vi "SerialMgr.vi"(0 "VISA Resource Name":refnum<visa-resource-name>="COM1", 1 "baud rate (921600)":u32=921600, 2 "data bits (8)":u16=8 min=5 max=8 step=1, 3 "parity (0:none)":enum16{"None", "Odd", "Even", "Mark", "Space"}(ring), 4 "stop bits (10: 1 bit)":u16(ring)=10 items=["1.0"=10, "1.5"=15, "2.0"=20], 5 "flow control (0:None)":enum16{"None", "XON/XOFF", "RTS/CTS"}(ring)) -> ()   [LabVIEW 2016]
doc: "This VI is the solution to Exercise 9-5 of the LabVIEW Basics I Course.\n\nThis VI communicates through the serial port to the NI Instrument Simulator using the VISA functions."
uses:
  SndMsgType.ctl
  <vilib>/Instr/_visa.llb/VISA Configure Serial Port (Instr).vi
  GlobalVars.vi
panel:
  # "* VISA resource name control *"
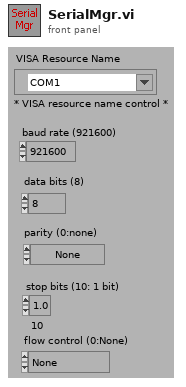
[diagram p1: front panel]
types:
  T1 = typedef "SndMsgType.ctl" = cluster{"Length":u16, "Formatted Msg":u8[]}
  T2 = typedef "Queue RefNum" = refnum<k1>
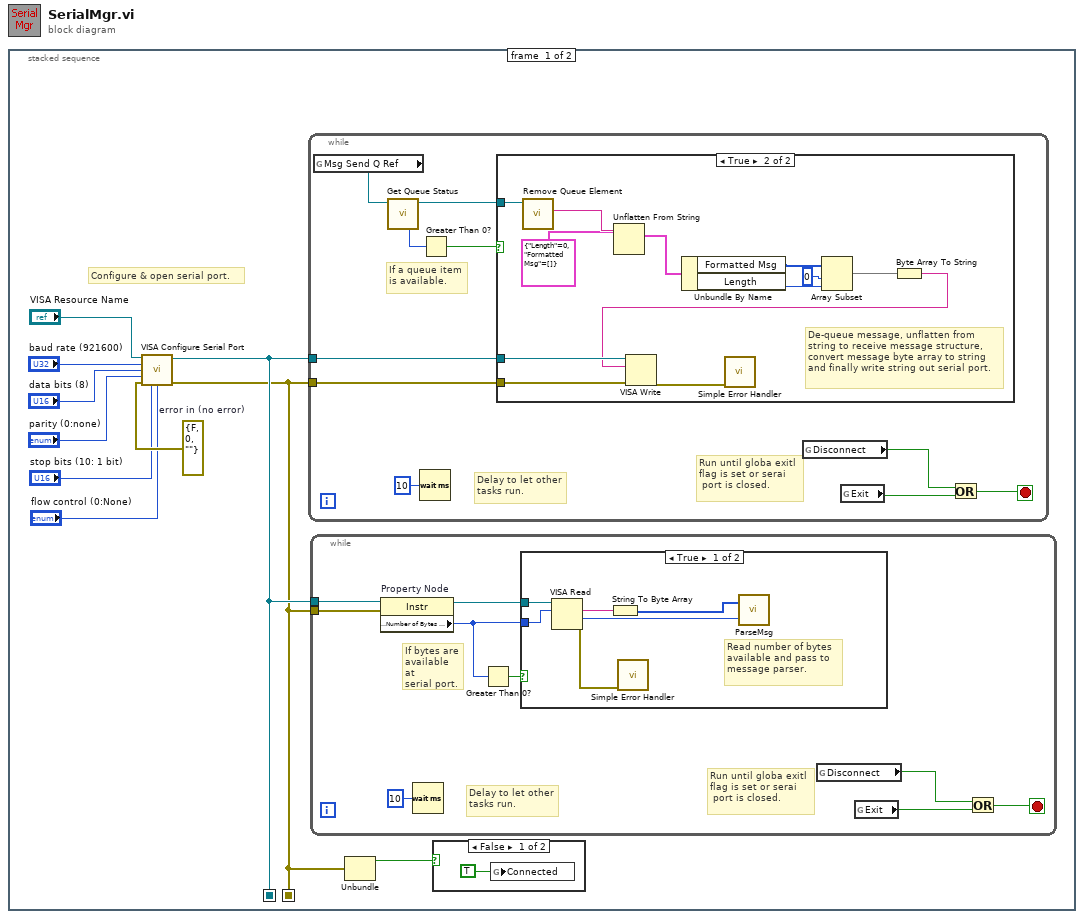
[diagram p0: block diagram]
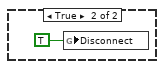
[diagram p2: hidden frame]
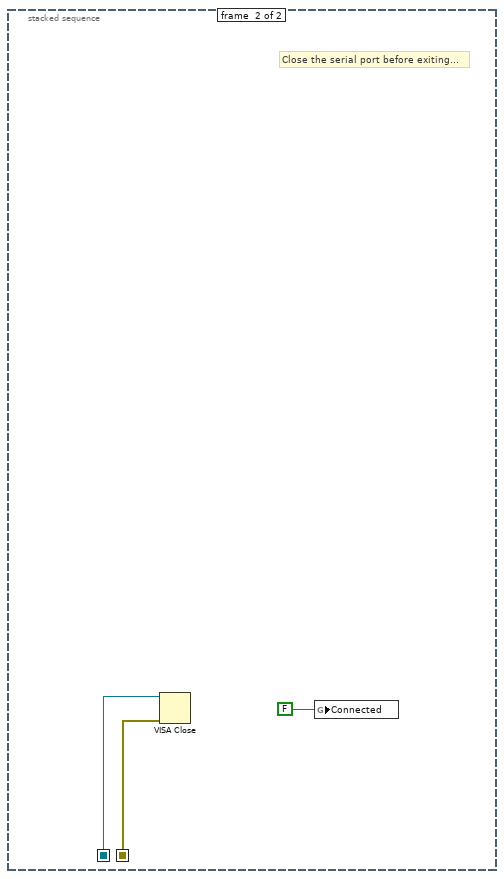
[diagram p5: hidden frame]
diagram:
  n1 = stacked-sequence {
    seq-local: [w2 _] -> [_ w52]
    seq-local: [w3 _] -> [_ w51]
    frame #0 {
      w9 = errorcluster {"status"=FALSE, "code"=0, "source"=""}  # error in (no error)
      # "Configure & open serial port."
      n2 = call-poly "VISA Configure Serial Port"("VISA resource name"="VISA Resource Name", "baud rate (9600)"="baud rate (921600)", "data bits (8)"="data bits (8)", "parity (0:none)"="parity (0:none)", "error in (no error)"=w9, "stop bits (10: 1 bit)"="stop bits (10: 1 bit)", "flow control (0:none)"="flow control (0:None)") -> ("VISA resource name out"=w3:refnum<visa-resource-name>, "error out"=w2:errorcluster)  [unwired: 7 in]
      n3 = while {
        tunnel: w3 -> [w37]
        tunnel: w2 -> [w36]
        stop <- w28 stop-if-true
        # "Delay to let other\ntasks run."
        # "Run until globa exitl\nflag is set or serai\n port is closed."
        # "If a queue item\nis available."
        n4 = global read "GlobalVars.vi" "Msg Send Q Ref"() -> (w34:T2)
        n5 = call <vilib>:"Get Queue Status.vi"("queue"=w34) -> ("queue out"=w31:T2, "# elements in queue"=w33:i32)  [unwired: 3 in, 6 out]
        n6 = Wait (ms)(milliseconds to wait=u32 10 ("millisecond multiple")) -> ()  [unwired: 1 out]
        n7 = Greater Than 0?(x=w33) -> (x > 0?=w32:bool)
        n8 = case shown="True" w32 {
          tunnel: w37 -> [_ w48]
          tunnel: w36 -> [_ w47]
          tunnel: w31 -> [_ w46]
          frame False {
          }
          frame True {
            # "De-queue message, unflatten from\nstring to receive message structure,\nconvert message byte array to string\nand finally write string out serial port."
            n9 = call <vilib>:"Remove Queue Element.vi"("queue"=w46) -> ("queue element"=w45:string)  [unwired: 5 in, 3 out]
            n10 = Unflatten From String(type=T1 {"Length"=0, "Formatted Msg"=[]} ("Snd Msg Type"), binary string=w45) -> (value=w43:T1)  [unwired: 3 in, 2 out]
            n11 = Unbundle By Name "Unbundle By Name"(w43) -> ("Formatted Msg"=w42:u8[], "Length"=w41:u16)
            n12 = Array Subset "Array Subset"(array=w42, index=0 ("Array Index"), length=w41) -> (w39:u8[])
            n13 = Byte Array To String(unsigned byte array=w39) -> (string=w38:string)
            n14 = VISA Write(VISA resource name=w48, write buffer=w38, error in (no error)=w47) -> (error out=w49:errorcluster)  [unwired: 2 out]
            n15 = call <vilib>:"Simple Error Handler.vi"("error in (no error)"=w49) -> ()  [unwired: 4 in, 5 out]
          }
        }
        n16 = global read "GlobalVars.vi" "Disconnect"() -> (w29:bool)
        n17 = global read "GlobalVars.vi" "Exit"() -> (w30:bool)
        n18 = Or(x=w29, y=w30) -> (x .or. y?=w28:bool)
      }
      n19 = while {
        tunnel: w2 -> [w19]
        tunnel: w3 -> [w20]
        stop <- w13 stop-if-true
        # "Run until globa exitl\nflag is set or serai\n port is closed."
        # "If bytes are\navailable at\nserial port."
        # "Delay to let other\ntasks run."
        n20 = property on="Property Node" class="Instr"(reference=w20, error in=w19) -> (reference out=w17:refnum<visa-resource-name>, "Serial Settings:Number of Bytes at Serial Port"=w16:u32)  [unwired: 1 out]
        n21 = Wait (ms)(milliseconds to wait=u32 10) -> ()  [unwired: 1 out]
        n22 = Greater Than 0?(x=w16) -> (x > 0?=w18:bool)
        n23 = case shown="True" w18 {
          tunnel: w16 -> [w26 _]
          tunnel: w17 -> [w25 _]
          frame True {
            # "Read number of bytes\navailable and pass to\nmessage parser."
            n24 = VISA Read(VISA resource name=w25, byte count=w26) -> (read buffer=w23:string, return count=w24:u32, error out=w27:errorcluster)  [unwired: 1 in, 1 out]
            n25 = String To Byte Array(string=w23) -> (unsigned byte array=w22:u8[])
            n26 = call <vilib>:"Simple Error Handler.vi"("error in (no error)"=w27) -> ()  [unwired: 4 in, 5 out]
            n27 = call "ParseMsg.vi"("Buf Len"=w24, "Input Buffer"=w22) -> ()  [unwired: 2 in]
          }
          frame False {
          }
        }
        n28 = global read "GlobalVars.vi" "Disconnect"() -> (w14:bool)
        n29 = global read "GlobalVars.vi" "Exit"() -> (w15:bool)
        n30 = Or(x=w14, y=w15) -> (x .or. y?=w13:bool)
      }
      n31 = Unbundle "Unbundle"(w2) -> ("status"=w1:bool)  [unwired: 2 out]
      n32 = case shown="False" w1 {
        frame False {
          n33 = global write "GlobalVars.vi" "Connected"(TRUE ("Connected")) -> ()
        }
        frame True {
          n34 = global write "GlobalVars.vi" "Disconnect"(TRUE ("Disconnect")) -> ()
        }
      }
    }
    frame #1 {
      # "Close the serial port before exiting..."
      n35 = VISA Close(VISA resource name=w51, error in (no error)=w52) -> ()  [unwired: 1 out]
      n36 = global write "GlobalVars.vi" "Connected"(FALSE ("Connected")) -> ()
    }
  }
